vi "User msg.vi"   [LabVIEW 2011]
uses:
  <vilib>/Rock Robotics/WPI/DriverStation/DriverStationLCD/WPI_DriverStationLCDLCDLine.ctl
  Robot Global Data.vi
types:
  T1 = typedef "WPI_DriverStationLCDLCDLine.ctl" = enum16{"Main - Line 1", "User - Line 2", "User - Line 3", "User - Line 4", "User - Line 5", "User - Line 6"}
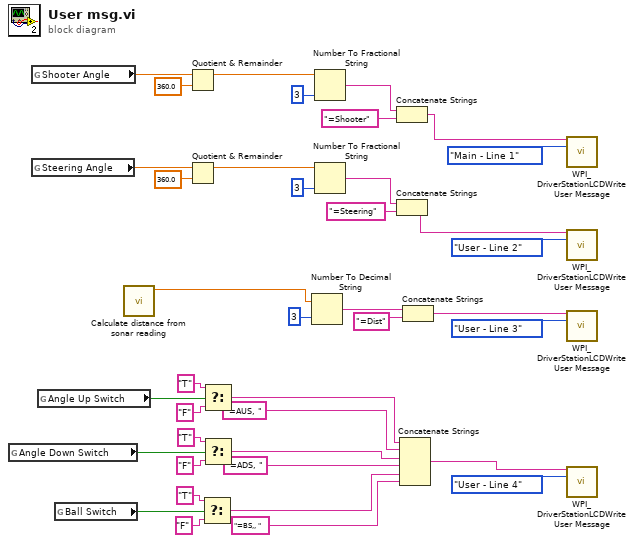
[diagram p0: block diagram]
diagram:
  n1 = global read "Robot Global Data.vi" "Angle Down Switch"() -> (w11:bool)
  n2 = global read "Robot Global Data.vi" "Shooter Angle"() -> (w29:dbl)
  n3 = global read "Robot Global Data.vi" "Steering Angle"() -> (w19:dbl)
  n4 = global read "Robot Global Data.vi" "Angle Up Switch"() -> (w14:bool)
  n5 = global read "Robot Global Data.vi" "Ball Switch"() -> (w8:bool)
  n6 = call "Calculate distance from sonar reading.vi"() -> ("Numeric"=w28:dbl)  [unwired: 11 in]
  n7 = Quotient & Remainder(x=w29, y=360.0) -> (x-y*floor(x/y)=w31:dbl)  [unwired: 1 out]
  n8 = Quotient & Remainder(x=w19, y=360.0) -> (x-y*floor(x/y)=w21:dbl)  [unwired: 1 out]
  n9 = Select(t="T", s=w8, f="F") -> (s? t:f=w3:string)
  n10 = Select(t="T", s=w14, f="F") -> (s? t:f=w1:string)
  n11 = Select(t="T", s=w11, f="F") -> (s? t:f=w5:string)
  n12 = Number To Decimal String(number=w28, width (-)=i16 3) -> (decimal integer string=w36:string)
  n13 = Number To Fractional String(number=w31, precision (6)=i16 3) -> (F-format string=w32:string)  [unwired: 2 in]
  n14 = Number To Fractional String(number=w21, precision (6)=i16 3) -> (F-format string=w22:string)  [unwired: 2 in]
  n15 = Concatenate Strings(w32, "=Shooter" ("string")) -> (w34:string)
  n16 = Concatenate Strings(w22, "=Steering" ("string")) -> (w24:string)
  n17 = Concatenate Strings(w1, "=AUS, " ("string"), w5, "=ADS, " ("string"), w3, "=BS,, " ("string")) -> (w16:string)
  n18 = Concatenate Strings(w36, "=Dist" ("string")) -> (w38:string)
  n19 = call <vilib>:"WPI_DriverStationLCDWrite User Message.vi"("line text"=w34, "line"=WPI_DriverStationLCDLCDLine."Main - Line 1") -> ()  [unwired: 13 in, 1 out]
  n20 = call <vilib>:"WPI_DriverStationLCDWrite User Message.vi"("line text"=w24, "line"=WPI_DriverStationLCDLCDLine."User - Line 2") -> ()  [unwired: 13 in, 1 out]
  n21 = call <vilib>:"WPI_DriverStationLCDWrite User Message.vi"("line text"=w38, "line"=WPI_DriverStationLCDLCDLine."User - Line 3") -> ()  [unwired: 13 in, 1 out]
  n22 = call <vilib>:"WPI_DriverStationLCDWrite User Message.vi"("line text"=w16, "line"=WPI_DriverStationLCDLCDLine."User - Line 4") -> ()  [unwired: 13 in, 1 out]
